vi "DistanceBetweenPoints.vi"(1 "coordinate 2\nnorth":dbl, 2 "coordinate 2\neast":dbl, 3 "coordinate 1\nnorth":dbl, 4 "coordinate 1\neast":dbl) -> (0 "Numeric":dbl)   [LabVIEW 2012]
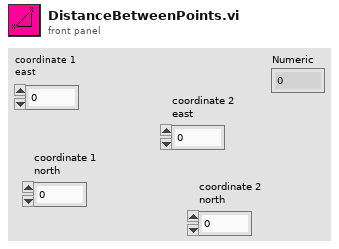
[diagram p1: front panel]
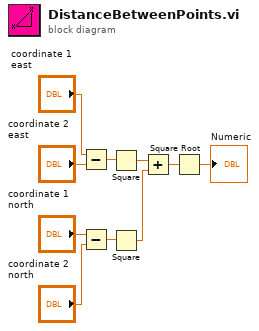
[diagram p0: block diagram]
diagram:
  n1 = Subtract(x="coordinate 1\neast", y="coordinate 2\neast") -> (x-y=w6:dbl)
  n2 = Subtract(x="coordinate 1\nnorth", y="coordinate 2\nnorth") -> (x-y=w5:dbl)
  n3 = Square(x=w6) -> (x^2=w7:dbl)
  n4 = Square(x=w5) -> (x^2=w8:dbl)
  n5 = Add(x=w7, y=w8) -> (x+y=w9:dbl)
  n6 = Square Root(x=w9) -> (sqrt(x)=→"Numeric":dbl)
